vi "rszvl_core_global.vi"() -> ()   [LabVIEW 2014] (continued)
Callback"="", "Coerce Callback"="", "User Callback"="", "Supported Models"="", "Instrument Options"="", "Repeated Capabilities"="", "Restricted Repeated Capabilities"="", "Help"="This attribute configures the R&S FSQ-K91 measurement type to be EVM Versus Carrier. After this command has been executed, the specified measurement will only be started when the user issues the INITiate command.\n\nAvailable Repeated Capabilities:\nNone\n\nRemote-control command(s):\nCONFigure:BURSt:EVM:ECARrier[:IMMediate]", "Flags"={"OPC Wait"=TRUE, "Dont check status"=FALSE, "*WAI"=FALSE}, "Check Status Callback"=""}, {"Level"=3, "Descriptive Name"="WLAN EVM Versus Symbol Measurement", "Class Only"=FALSE, "Data Type"=4, "Access"=1, "Identifier"="RSZVL_ATTR_WLAN_EVM_ESYM", "Range Table"="", "Command"="CONF:BURS:EVM:ESYM", "Read Callback"="", "Write Callback"="", "Range Callback"="", "Check Callback"="", "Rngtable Callback"="", "Coerce Callback"="", "User Callback"="", "Supported Models"="", "Instrument Options"="", "Repeated Capabilities"="", "Restricted Repeated Capabilities"="", "Help"="This attribute configures the FSQ-K91 measurement type to be EVM Versus Symbol. After this command has been executed, the specified measurement will only be started when the user issues the INITiate command\n\nAvailable Repeated Capabilities:\nNone\n\nRemote-control command(s):\nCONFigure:BURSt:EVM:ESYMbol[:IMMediate]", "Flags"={"OPC Wait"=TRUE, "Dont check status"=FALSE, "*WAI"=FALSE}, "Check Status Callback"=""}, {"Level"=3, "Descriptive Name"="WLAN Spectrum MASK", "Class Only"=FALSE, "Data Type"=4, "Access"=1, "Identifier"="RSZVL_ATTR_WLAN_SPEC_MASK", "Range Table"="", "Command"="CONF:BURS:SPEC:MASK", "Read Callback"="", "Write Callback"="", "Range Callback"="", "Check Callback"="", "Rngtable Callback"="", "Coerce Callback"="", "User Callback"="", "Supported Models"="", "Instrument Options"="", "Repeated Capabilities"="", "Restricted Repeated Capabilities"="", "Help"="This attribute configures the R&S FSQ-K91 measurement type to be Spectrum mask. After this command has been executed, the specified measurement will only be started when the user issues the INITiate command\n\nAvailable Repeated Capabilities:\nNone\n\nRemote-control command(s):\nCONFigure:BURSt:SPECtrum:MASK[:IMMediate]", "Flags"={"OPC Wait"=TRUE, "Dont check status"=FALSE, "*WAI"=FALSE}, "Check Status Callback"=""}, {"Level"=3, "Descriptive Name"="WLAN Spectrum MASK Select", "Class Only"=FALSE, "Data Type"=0, "Access"=2, "Identifier"="RSZVL_ATTR_WLAN_SPEC_MASK_SEL", "Range Table"="rszvl_rngSpecMask", "Command"="CONF:BURS:SPEC:MASK:SEL", "Read Callback"="", "Write Callback"="", "Range Callback"="", "Check Callback"="", "Rngtable Callback"="", "Coerce Callback"="", "User Callback"="", "Supported Models"="", "Instrument Options"="", "Repeated Capabilities"="", "Restricted Repeated Capabilities"="", "Help"="This attribute configures how R&S FS-K91 will interpret the Spectrum MASK measurement results.\nThis is either performed using the IEEE or ETSI standard. \n\nNote:\n(1) This attribute is only available for IEEE\n802.11a.\n\nAvailable Repeated Capabilities:\nNone\n\nRemote-control command(s):\nCONFigure:BURSt:SPECtrum:MASK:SELect IEEE | ETSI", "Flags"={"OPC Wait"=FALSE, "Dont check status"=FALSE, "*WAI"=FALSE}, "Check Status Callback"=""}, {"Level"=3, "Descriptive Name"="WLAN Spectrum FFT", "Class Only"=FALSE, "Data Type"=4, "Access"=1, "Identifier"="RSZVL_ATTR_WLAN_SPEC_FFT", "Range Table"="", "Command"="CONF:BURS:SPEC:FFT", "Read Callback"="", "Write Callback"="", "Range Callback"="", "Check Callback"="", "Rngtable Callback"="", "Coerce Callback"="", "User Callback"="", "Supported Models"="", "Instrument Options"="", "Repeated Capabilities"="", "Restricted Repeated Capabilities"="", "Help"="This attribute configures the R&S FSQ-K91 measurement type to be FFT (Fast Fourier Transform). After this command has been executed, the specified measurement will only be started when the user issues the INITiate command\n\nAvailable Repeated Capabilities:\nNone\n\nRemote-control command(s):\nCONFigure:BURSt:SPECtrum:FFT[:IMMediate]", "Flags"={"OPC Wait"=TRUE, "Dont check status"=FALSE, "*WAI"=FALSE}, "Check Status Callback"=""}, {"Level"=3, "Descriptive Name"="WLAN Spectrum ACPR", "Class Only"=FALSE, "Data Type"=4, "Access"=1, "Identifier"="RSZVL_ATTR_WLAN_SPEC_ACPR", "Range Table"="", "Command"="CONF:BURS:SPEC:ACPR", "Read Callback"="", "Write Callback"="", "Range Callback"="", "Check Callback"="", "Rngtable Callback"="", "Coerce Callback"="", "User Callback"="", "Supported Models"="", "Instrument Options"="", "Repeated Capabilities"="", "Restricted Repeated Capabilities"="", "Help"="This attribute configures the R&S FSQ-K91/K92 measurement type to be ACPR (adjacent channel power ratio). After this command has been executed, the specified measurement will only be started when the user issues the INITiate command\n\nAvailable Repeated Capabilities:\nNone\n\nRemote-control command(s):\nCONFigure:BURSt:SPECtrum:ACPR[:IMMediate]", "Flags"={"OPC Wait"=TRUE, "Dont check status"=FALSE, "*WAI"=FALSE}, "Check Status Callback"=""}, {"Level"=3, "Descriptive Name"="WLAN Constelation Versus Symbol", "Class Only"=FALSE, "Data Type"=4, "Access"=1, "Identifier"="RSZVL_ATTR_WLAN_CONS_CSYM", "Range Table"="", "Command"="CONF:BURS:CONS:CSYM", "Read Callback"="", "Write Callback"="", "Range Callback"="", "Check Callback"="", "Rngtable Callback"="", "Coerce Callback"="", "User Callback"="", "Supported Models"="", "Instrument Options"="", "Repeated Capabilities"="", "Restricted Repeated Capabilities"="", "Help"="This attribute configures the R&S FSQ-K91 measurement type to be Constellation versus Symbol. After this command has been executed, the specified measurement will only be started when the user issues the INITiate command\n\nAvailable Repeated Capabilities:\nNone\n\nRemote-control command(s):\nCONFigure:BURSt:CONStellation:CSYMbol[:IMMediate]", "Flags"={"OPC Wait"=TRUE, "Dont check status"=FALSE, "*WAI"=FALSE}, "Check Status Callback"=""}, {"Level"=3, "Descriptive Name"="WLAN Overall Burst Count", "Class Only"=FALSE, "Data Type"=3, "Access"=2, "Identifier"="RSZVL_ATTR_WLAN_BURS_COUN_STAT", "Range Table"="", "Command"="BURS:COUN:STAT", "Read Callback"="", "Write Callback"="", "Range Callback"="", "Check Callback"="", "Rngtable Callback"="", "Coerce Callback"="", "User Callback"="", "Supported Models"="", "Instrument Options"="", "Repeated Capabilities"="", "Restricted Repeated Capabilities"="", "Help"="When this attribute is set to on, the burst count parameter will be used by the measurement,\notherwise the burst count parameter will be ignored.\n\nAvailable Repeated Capabilities:\nNone\n\nRemote-control command(s):\n[SENSe:]BURSt:COUNt:STATe ON | OFF", "Flags"={"OPC Wait"=FALSE, "Dont check status"=FALSE, "*WAI"=FALSE}, "Check Status Callback"=""}, {"Level"=3, "Descriptive Name"="WLAN Constelation Versus Carrier", "Class Only"=FALSE, "Data Type"=4, "Access"=1, "Identifier"="RSZVL_ATTR_WLAN_CONS_CCAR", "Range Table"="", "Command"="CONF:BURS:CONS:CCAR", "Read Callback"="", "Write Callback"="", "Range Callback"="", "Check Callback"="", "Rngtable Callback"="", "Coerce Callback"="", "User Callback"="", "Supported Models"="", "Instrument Options"="", "Repeated Capabilities"="", "Restricted Repeated Capabilities"="", "Help"="This attribute configures the R&S FSQ-K91 measurement type to be Constellation versus Carrier. After this command has been executed, the specified\nmeasurement will only be started when the user issues the INITiate command.\n\nAvailable Repeated Capabilities:\nNone\n\nRemote-control command(s):\nCONFigure:BURSt:CONStellation:CCARrier[:IMMediate]", "Flags"={"OPC Wait"=TRUE, "Dont check status"=FALSE, "*WAI"=FALSE}, "Check Status Callback"=""}, {"Level"=3, "Descriptive Name"="WLAN Constellation Carrier Select", "Class Only"=FALSE, "Data Type"=0, "Access"=2, "Identifier"="RSZVL_ATTR_WLAN_CONS_CARR_SEL", "Range Table"="rszvl_rngBurstSel", "Command"="CONF:BURS:CONS:CARR:SEL", "Read Callback"="", "Write Callback"="", "Range Callback"="", "Check Callback"="", "Rngtable Callback"="", "Coerce Callback"="", "User Callback"="", "Supported Models"="", "Instrument Options"="", "Repeated Capabilities"="", "Restricted Repeated Capabilities"="", "Help"="This attribute is only available when Constellation versus Symbol measurement is selected. When the Constellation versus Symbol measurement is initiated, it will calculate the results of the selected carrier.\n\nNote:\n(1) This attribute is not available for IEEE 802.11b standard.\n\nAvailable Repeated Capabilities:\nNone\n\nRemote-control command(s):\nCONFigure:BURSt:CONStellation:CARRier:SELect ALL | PILOTS", "Flags"={"OPC Wait"=FALSE, "Dont check status"=FALSE, "*WAI"=FALSE}, "Check Status Callback"=""}, {"Level"=3, "Descriptive Name"="WLAN Constellation Carrier Select Num", "Class Only"=FALSE, "Data Type"=0, "Access"=2, "Identifier"="RSZVL_ATTR_WLAN_CONS_CARR_SEL_NR", "Range Table"="", "Command"="CONF:BURS:CONS:CARR:SEL", "Read Callback"="", "Write Callback"="", "Range Callback"="", "Check Callback"="", "Rngtable Callback"="", "Coerce Callback"="", "User Callback"="", "Supported Models"="", "Instrument Options"="", "Repeated Capabilities"="", "Restricted Repeated Capabilities"="", "Help"="This attribute is only available when Constellation versus Symbol measurement is selected. When the Constellation versus Symbol measurement is initiated, it will calculate the results of the selected carrier.\n\nNote:¨\n(1) This attribute is not available for IEEE 802.11b standard.\n\n(2) Values -26 to 26 exclude 0 are available\n\nAvailable Repeated Capabilities:\nNone\n\nRemote-control command(s):\nCONFigure:BURSt:CONStellation:CARRier:SELect nr", "Flags"={"OPC Wait"=FALSE, "Dont check status"=FALSE, "*WAI"=FALSE}, "Check Status Callback"=""}, {"Level"=3, "Descriptive Name"="WLAN Statistics CCDF", "Class Only"=FALSE, "Data Type"=4, "Access"=1, "Identifier"="RSZVL_ATTR_WLAN_STAT_CCDF", "Range Table"="", "Command"="CONF:BURS:STAT:CCDF", "Read Callback"="", "Write Callback"="", "Range Callback"="", "Check Callback"="", "Rngtable Callback"="", "Coerce Callback"="", "User Callback"="", "Supported Models"="", "Instrument Options"="", "Repeated Capabilities"="", "Restricted Repeated Capabilities"="", "Help"="This attribute configures the R&S FSQ-K91 measurement type to be CCDF (conditional cumulative distribution functions.). After this command has been executed, the specified measurement will only be started when the user issues the INITiate command\n\nAvailable Repeated Capabilities:\nNone\n\nRemote-control command(s):\nCONFigure:BURSt:STATistics:CCDF[:IMMediate]", "Flags"={"OPC Wait"=TRUE, "Dont check status"=FALSE, "*WAI"=FALSE}, "Check Status Callback"=""}, {"Level"=3, "Descriptive Name"="WLAN Statistics Bit Stream", "Class Only"=FALSE, "Data Type"=4, "Access"=1, "Identifier"="RSZVL_ATTR_WLAN_STAT_BSTR", "Range Table"="", "Command"="CONF:BURS:STAT:BSTR", "Read Callback"="", "Write Callback"="", "Range Callback"="", "Check Callback"="", "Rngtable Callback"="", "Coerce Callback"="", "User Callback"="", "Supported Models"="", "Instrument Options"="", "Repeated Capabilities"="", "Restricted Repeated Capabilities"="", "Help"="This attribute configures the R&S FSQ-K91 measurement type to be bit stream. After this command has been executed, the specified measurement will only be started when the user issues the INITiate command\n\nAvailable Repeated Capabilities:\nNone\n\nRemote-control command(s):\nCONFigure:BURSt:STATistics:BSTReam[:IMMediate]", "Flags"={"OPC Wait"=TRUE, "Dont check status"=FALSE, "*WAI"=FALSE}, "Check Status Callback"=""}, {"Level"=3, "Descriptive Name"="WLAN Statistics Signal Field", "Class Only"=FALSE, "Data Type"=4, "Access"=1, "Identifier"="RSZVL_ATTR_WLAN_STAT_SFI", "Range Table"="", "Command"="CONF:BURS:STAT:SFI", "Read Callback"="", "Write Callback"="", "Range Callback"="", "Check Callback"="", "Rngtable Callback"="", "Coerce Callback"="", "User Callback"="", "Supported Models"="", "Instrument Options"="", "Repeated Capabilities"="", "Restricted Repeated Capabilities"="", "Help"="This attribute configures the R&S FS-K91 measurement type to be signal field. After this command has been executed, the specified measurement will only be started when the user issues the INITiate command.\n\nAvailable Repeated Capabilities:\nNone\n\nRemote-control command(s):\nCONFigure:BURSt:STATistics:SFIeld [:IMMediate]", "Flags"={"OPC Wait"=TRUE, "Dont check status"=FALSE, "*WAI"=FALSE}, "Check Status Callback"=""}, {"Level"=3, "Descriptive Name"="WLAN Start Measurement", "Class Only"=FALSE, "Data Type"=4, "Access"=1, "Identifier"="RSZVL_ATTR_WLAN_INIT", "Range Table"="", "Command"="INIT", "Read Callback"="", "Write Callback"="", "Range Callback"="", "Check Callback"="", "Rngtable Callback"="", "Coerce Callback"="", "User Callback"="", "Supported Models"="", "Instrument Options"="", "Repeated Capabilities"="", "Restricted Repeated Capabilities"="", "Help"="This attribute requests the R&S FSQ-K91 option to start a new measurement sequence. If a measurement sequence is already in progress, the command will be ignored.\n\nAvailable Repeated Capabilities:\nNone\n\nRemote-control command(s):\nINITiate[:IMMediate]", "Flags"={"OPC Wait"=TRUE, "Dont check status"=FALSE, "*WAI"=FALSE}, "Check Status Callback"=""}, {"Level"=3, "Descriptive Name"="WLAN Run Continuous", "Class Only"=FALSE, "Data Type"=3, "Access"=2, "Identifier"="RSZVL_ATTR_WLAN_INIT_CONT", "Range Table"="", "Command"="INIT:CONT", "Read Callback"="", "Write Callback"="", "Range Callback"="", "Check Callback"="", "Rngtable Callback"="", "Coerce Callback"="", "User Callback"="", "Supported Models"="", "Instrument Options"="", "Repeated Capabilities"="", "Restricted Repeated Capabilities"="", "Help"="This attribute determines whether the trigger system is continuously initiated (continuous) or\nperforms single measurements (single).\n\nAvailable Repeated Capabilities:\nNone\n\nRemote-control command(s):\nINITiate:CONTinuous ON | OFF", "Flags"={"OPC Wait"=FALSE, "Dont check status"=FALSE, "*WAI"=FALSE}, "Check Status Callback"=""}, {"Level"=3, "Descriptive Name"="WLAN Mode", "Class Only"=FALSE, "Data Type"=4, "Access"=1, "Identifier"="RSZVL_ATTR_WLAN_MODE", "Range Table"="", "Command"="INST:SEL WLAN", "Read Callback"="", "Write Callback"="", "Range Callback"="", "Check Callback"="", "Rngtable Callback"="", "Coerce Callback"="", "User Callback"="", "Supported Models"="", "Instrument Options"="", "Repeated Capabilities"="", "Restricted Repeated Capabilities"="", "Help"="This attribute selects active operation of the R&S FSQ-K91 option by specifying its name.\n\nAvailable Repeated Capabilities:\nNone\n\nRemote-control command(s):\nINSTrument:SELect WLAN", "Flags"={"OPC Wait"=FALSE, "Dont check status"=FALSE, "*WAI"=FALSE}, "Check Status Callback"=""}, {"Level"=3, "Descriptive Name"="WLAN Number of Burst", "Class Only"=FALSE, "Data Type"=0, "Access"=2, "Identifier"="RSZVL_ATTR_WLAN_BURS_COUN", "Range Table"="", "Command"="BURS:COUN", "Read Callback"="", "Write Callback"="", "Range Callback"="", "Check Callback"="", "Rngtable Callback"="", "Coerce Callback"="", "User Callback"="", "Supported Models"="", "Instrument Options"="", "Repeated Capabilities"="", "Restricted Repeated Capabilities"="", "Help"="This attribute defines the number of bursts that will be analyzed by the measurement. This attribute is not valid, if the setting for the [SENSe:]BURst:COUNt:STATe parameter is off.\n\nAvailable Repeated Capabilities:\nNone\n\nRemote-control command(s):\n[SENSe:]BURSt:COUNt", "Flags"={"OPC Wait"=FALSE, "Dont check status"=FALSE, "*WAI"=FALSE}, "Check Status Callback"=""}, {"Level"=3, "Descriptive Name"="WLAN Swap IQ", "Class Only"=FALSE, "Data Type"=3, "Access"=2, "Identifier"="RSZVL_ATTR_WLAN_SWAP_IQ", "Range Table"="", "Command"="SWAP", "Read Callback"="", "Write Callback"="", "Range Callback"="", "Check Callback"="", "Rngtable Callback"="", "Coerce Callback"="", "User Callback"="", "Supported Models"="", "Instrument Options"="", "Repeated Capabilities"="", "Restricted Repeated Capabilities"="", "Help"="This attribute defines whether or not the recorded IQ pairs should be swapped (I/Q) before being processed.\n\nAvailable Repeated Capabilities:\nNone\n\nRemote-control command(s):\n[SENSe:]SWAPiq ON|OFF", "Flags"={"OPC Wait"=FALSE, "Dont check status"=FALSE, "*WAI"=FALSE}, "Check Status Callback"=""}, {"Level"=3, "Descriptive Name"="WLAN ACP Mode", "Class Only"=FALSE, "Data Type"=0, "Access"=2, "Identifier"="RSZVL_ATTR_WLAN_ACH_MODE", "Range Table"="rszvl_rngAbsRel", "Command"="POW:ACH:MODE", "Read Callback"="", "Write Callback"="", "Range Callback"="", "Check Callback"="", "Rngtable Callback"="", "Coerce Callback"="", "User Callback"="", "Supported Models"="", "Instrument Options"="", "Repeated Capabilities"="", "Restricted Repeated Capabilities"="", "Help"="This attribut sets the ACP measurement mode to either absolute or relative.\n\nNote:\n(1) This attribute is available only for IEEE 802.11j standard.\n\nAvailable Repeated Capabilities:\nNone\n\nRemote-control command(s):\n[SENSe:]POWer:ACHannel:MODE ABS | REL", "Flags"={"OPC Wait"=FALSE, "Dont check status"=FALSE, "*WAI"=FALSE}, "Check Status Callback"=""}, {"Level"=3, "Descriptive Name"="WLAN Preamble Unit", "Class Only"=FALSE, "Data Type"=0, "Access"=2, "Identifier"="RSZVL_ATTR_WLAN_UNIT_PRE", "Range Table"="rszvl_rngUnitHzPct", "Command"="UNIT:PRE", "Read Callback"="", "Write Callback"="", "Range Callback"="", "Check Callback"="", "Rngtable Callback"="", "Coerce Callback"="", "User Callback"="", "Supported Models"="", "Instrument Options"="", "Repeated Capabilities"="", "Restricted Repeated Capabilities"="", "Help"="This attribute specifies the units for Preamble error results.\n\nAvailable Repeated Capabilities:\nNone\n\nRemote-control command(s):\nUNIT:PREamble HZ | PCT", "Flags"={"OPC Wait"=FALSE, "Dont check status"=FALSE, "*WAI"=FALSE}, "Check Status Callback"=""}, {"Level"=3, "Descriptive Name"="WLAN EVM Unit", "Class Only"=FALSE, "Data Type"=0, "Access"=2, "Identifier"="RSZVL_ATTR_WLAN_UNIT_EVM", "Range Table"="rszvl_rngUnitDbPct", "Command"="UNIT:EVM", "Read Callback"="", "Write Callback"="", "Range Callback"="", "Check Callback"="", "Rngtable Callback"="", "Coerce Callback"="", "User Callback"="", "Supported Models"="", "Instrument Options"="", "Repeated Capabilities"="", "Restricted Repeated Capabilities"="", "Help"="This attribute specifies the units for EVM trace results.\n\nAvailable Repeated Capabilities:\nNone\n\nRemote-control command(s):\nUNIT:EVM DB | PCT", "Flags"={"OPC Wait"=FALSE, "Dont check status"=FALSE, "*WAI"=FALSE}, "Check Status Callback"=""}, {"Level"=3, "Descriptive Name"="WLAN Gain Imbalance Unit", "Class Only"=FALSE, "Data Type"=0, "Access"=2, "Identifier"="RSZVL_ATTR_WLAN_UNIT_GIMB", "Range Table"="rszvl_rngUnitDbPct", "Command"="UNIT:GIMBalance", "Read Callback"="", "Write Callback"="", "Range Callback"="", "Check Callback"="", "Rngtable Callback"="", "Coerce Callback"="", "User Callback"="", "Supported Models"="", "Instrument Options"="", "Repeated Capabilities"="", "Restricted Repeated Capabilities"="", "Help"="This attribute specifies the units for gain imbalance results.\n\nAvailable Repeated Capabilities:\nNone\n\nRemote-control command(s):\nUNIT:GIMBalance DB | PCT", "Flags"={"OPC Wait"=FALSE, "Dont check status"=FALSE, "*WAI"=FALSE}, "Check Status Callback"=""}, {"Level"=3, "Descriptive Name"="WLAN Phase or Frequency vs Preamble", "Class Only"=FALSE, "Data Type"=4, "Access"=1, "Identifier"="RSZVL_ATTR_WLAN_PRE", "Range Table"="", "Command"="CONF:BURS:PRE", "Read Callback"="", "Write Callback"="", "Range Callback"="", "Check Callback"="", "Rngtable Callback"="", "Coerce Callback"="", "User Callback"="", "Supported Models"="", "Instrument Options"="", "Repeated Capabilities"="", "Restricted Repeated Capabilities"="", "Help"="This attribute configures the R&S FSQ-K90/K91 measurement type to be Phase or Frequency Vs Premable. After this command has been executed, the specified measurement will only be started when the user issues the INITiate command\n\nAvailable Repeated Capabilities:\nNone\n\nRemote-control command(s):\nCONFigure:BURSt:PREamble[:IMMediate]", "Flags"={"OPC Wait"=FALSE, "Dont check status"=FALSE, "*WAI"=FALSE}, "Check Status Callback"=""}, {"Level"=3, "Descriptive Name"="WLAN IQ Sample Rate", "Class Only"=FALSE, "Data Type"=1, "Access"=2, "Identifier"="RSZVL_ATTR_WLAN_SRAT", "Range Table"="rszvl_rngIQSRate", "Command"="TRACE:IQ:SRAT", "Read Callback"="", "Write Callback"="", "Range Callback"="", "Check Callback"="", "Rngtable Callback"="", "Coerce Callback"="", "User Callback"="", "Supported Models"="", "Instrument Options"="", "Repeated Capabilities"="", "Restricted Repeated Capabilities"="", "Help"="This attribute allows the sample rate for IQ measurements to be specified. \n\nValid Range: 10.0e3 Hz to 100.0e6 Hz (326.4e6 Hz with option R&S FSQ-B72)\n\nAvailable Repeated Capabilities:\nNone\n\nRemote-control command(s):\nTRACE:IQ:SRATe", "Flags"={"OPC Wait"=FALSE, "Dont check status"=FALSE, "*WAI"=FALSE}, "Check Status Callback"=""}, {"Level"=3, "Descriptive Name"="WLAN Automatic Power Level Sweep Time", "Class Only"=FALSE, "Data Type"=1, "Access"=2, "Identifier"="RSZVL_ATTR_WLAN_POW_AUTO_SWE_TIME", "Range Table"="rszvl_rngAutoLevelTime", "Command"="CONF:POW:AUTO:SWE:TIME", "Read Callback"="", "Write Callback"="", "Range Callback"="", "Check Callback"="", "Rngtable Callback"="", "Coerce Callback"="", "User Callback"="", "Supported Models"="", "Instrument Options"="", "Repeated Capabilities"="", "Restricted Repeated Capabilities"="", "Help"="This attribute specifies the sweep time for the automatic power level detection.\n\nAvailable Repeated Capabilities:\nNone\n\nRemote-control command(s):\nCONFigure:POWer:AUTO:SWEep:TIME", "Flags"={"OPC Wait"=FALSE, "Dont check status"=FALSE, "*WAI"=FALSE}, "Check Status Callback"=""}, {"Level"=3, "Descriptive Name"="WLAN Load IQ Data", "Class Only"=FALSE, "Data Type"=2, "Access"=1, "Identifier"="RSZVL_ATTR_WLAN_IQ_LOAD", "Range Table"="", "Command"="MMEM:LOAD:IQ:STAT", "Read Callback"="", "Write Callback"="rszvl_FileStateSpecialFormat_WriteCallback.vi", "Range Callback"="", "Check Callback"="", "Rngtable Callback"="", "Coerce Callback"="", "User Callback"="", "Supported Models"="", "Instrument Options"="", "Repeated Capabilities"="", "Restricted Repeated Capabilities"="", "Help"="This attribute loads IQ data from the specified .iqw file.\n\nAvailable Repeated Capabilities:\nNone\n\nRemote-control command(s):\nMMEMory:LOAD:IQ:STATe", "Flags"={"OPC Wait"=FALSE, "Dont check status"=FALSE, "*WAI"=FALSE}, "Check Status Callback"=""}, {"Level"=3, "Descriptive Name"="WLAN Save IQ Data", "Class Only"=FALSE, "Data Type"=2, "Access"=1, "Identifier"="RSZVL_ATTR_WLAN_IQ_SAVE", "Range Table"="", "Command"="MMEM:STOR:IQ:STAT", "Read Callback"="", "Write Callback"="rszvl_FileStateSpecialFormat_WriteCallback.vi", "Range Callback"="", "Check Callback"="", "Rngtable Callback"="", "Coerce Callback"="", "User Callback"="", "Supported Models"="", "Instrument Options"="", "Repeated Capabilities"="", "Restricted Repeated Capabilities"="", "Help"="This attribute stores IQ data to the specified .iqw file.\n\nAvailable Repeated Capabilities:\nNone\n\nRemote-control command(s):\nMMEMory:STORe:IQ:STATe", "Flags"={"OPC Wait"=FALSE, "Dont check status"=FALSE, "*WAI"=FALSE}, "Check Status Callback"=""}, {"Level"=3, "Descriptive Name"="WLAN Burst Recalculate", "Class Only"=FALSE, "Data Type"=4, "Access"=1, "Identifier"="RSZVL_ATTR_WLAN_CALC_BURS", "Range Table"="", "Command"="CALC:BURS", "Read Callback"="", "Write Callback"="", "Range Callback"="", "Check Callback"="", "Rngtable Callback"="", "Coerce Callback"="", "User Callback"="", "Supported Models"="", "Instrument Options"="", "Repeated Capabilities"="", "Restricted Repeated Capabilities"="", "Help"="This attribute forces the IQ measurement results to be recalculated according to the current settings\n\nAvailable Repeated Capabilities:\nNone\n\nRemote-control command(s):\nCALCulate<1|2>:BURSt[:IMMediate]", "Flags"={"OPC Wait"=FALSE, "Dont check status"=FALSE, "*WAI"=FALSE}, "Check Status Callback"=""}, {"Level"=3, "Descriptive Name"="WLAN Preamble Select", "Class Only"=FALSE, "Data Type"=0, "Access"=2, "Identifier"="RSZVL_ATTR_WLAN_PRE_SEL", "Range Table"="rszvl_rngPreamble", "Command"="CONF:BURS:PRE:SEL", "Read Callback"="", "Write Callback"="", "Range Callback"="", "Check Callback"="", "Rngtable Callback"="", "Coerce Callback"="", "User Callback"="", "Supported Models"="", "Instrument Options"="", "Repeated Capabilities"="", "Restricted Repeated Capabilities"="", "Help"="This attribute specifies whether Frequency or Phase results are displayed when the\nmeasurement type is set to Error Vs Preamble\n\nAvailable Repeated Capabilities:\nNone\n\nRemote-control command(s):\nCONFigure:BURSt:PREamble:SELect FREQ | PHASe", "Flags"={"OPC Wait"=FALSE, "Dont check status"=FALSE, "*WAI"=FALSE}, "Check Status Callback"=""}, {"Level"=2, "Descriptive Name"="Display", "Class Only"=TRUE, "Data Type"=0, "Access"=0, "Identifier"="", "Range Table"="", "Command"="", "Read Callback"="", "Write Callback"="", "Range Callback"="", "Check Callback"="", "Rngtable Callback"="", "Coerce Callback"="", "User Callback"="", "Supported Models"="", "Instrument Options"="", "Repeated Capabilities"="", "Restricted Repeated Capabilities"="", "Help"="Attributes that configure the display.\n\n(1) WLAN Display Table:\nThis attribute selects whether the results table is displayed.\n\n(2) WLAN Y Axis Auto Scaling:\nThis attribute switches on or off automatic scaling of the Y-axis for the specified trace display. Automatic scaling sets the Y-axis to automatically scale to best fit the measurement results. \n\nNote:\n(1) This attribute is only available for the following result displays:\nEVM vs Carrier\nEVM vs Symbol\nFrequency error vs Preamble\nPhase error vs Preamble\n\n\n(3) WLAN Y Scale Division:\nThis attribute sets the size of each Y scale division for the specified trace display. \n\nNote:\n(1) This attribute has no affect if automatic scaling of the Y-axis is enabled. \n\n(2) This attribute is only available for\nthe following result displays:\nEVM vs Carrier\nEVM vs Symbol\nFrequency error vs Preamble\nPhase error vs Preamble", "Flags"={"OPC Wait"=FALSE, "Dont check status"=FALSE, "*WAI"=FALSE}, "Check Status Callback"=""}, {"Level"=3, "Descriptive Name"="WLAN Display Table", "Class Only"=FALSE, "Data Type"=3, "Access"=2, "Identifier"="RSZVL_ATTR_WLAN_DISP_TABL", "Range Table"="", "Command"="DISP:WIND:TABL", "Read Callback"="", "Write Callback"="", "Range Callback"="", "Check Callback"="", "Rngtable Callback"="", "Coerce Callback"="", "User Callback"="", "Supported Models"="", "Instrument Options"="", "Repeated Capabilities"="", "Restricted Repeated Capabilities"="", "Help"="This attribute selects whether the results table is displayed.\n\nAvailable Repeated Capabilities:\nNone\n\nRemote-control command(s):\nDISPlay[:WINDow<1|2>]:TABLe ON | OFF", "Flags"={"OPC Wait"=FALSE, "Dont check status"=FALSE, "*WAI"=FALSE}, "Check Status Callback"=""}, {"Level"=3, "Descriptive Name"="WLAN Screen Select", "Class Only"=FALSE, "Data Type"=4, "Access"=1, "Identifier"="RSZVL_ATTR_WLAN_SCREEN_SELECT", "Range Table"="", "Command"="DISP:WIND{Window}:SSEL", "Read Callback"="", "Write Callback"="", "Range Callback"="", "Check Callback"="", "Rngtable Callback"="", "Coerce Callback"="", "User Callback"="", "Supported Models"="", "Instrument Options"="", "Repeated Capabilities"="", "Restricted Repeated Capabilities"="", "Help"="This attribute selects whether screen A or screen B is active. SSELect means Screen SELect.\n\nAvailable Repeated Capabilities:\nWindow: Win1,Win2\r\n\nRemote-control command(s):\nDISPlay[:WINDow<1|2>]:SSELect", "Flags"={"OPC Wait"=FALSE, "Dont check status"=FALSE, "*WAI"=FALSE}, "Check Status Callback"=""}, {"Level"=3, "Descriptive Name"="WLAN Display Format", "Class Only"=FALSE, "Data Type"=0, "Access"=2, "Identifier"="RSZVL_ATTR_WLAN_DISP_FORMAT", "Range Table"="rszvl_rngDISPFormat", "Command"="DISP:FORM", "Read Callback"="", "Write Callback"="", "Range Callback"="", "Check Callback"="", "Rngtable Callback"="", "Coerce Callback"="", "User Callback"="", "Supported Models"="", "Instrument Options"="", "Repeated Capabilities"="", "Restricted Repeated Capabilities"="", "Help"="This attribute sets the visible screen display type to full or split screen.\n\nAvailable Repeated Capabilities:\nNone\n\nRemote-control command(s):\nDISPlay:FORMat SINGle | SPLit", "Flags"={"OPC Wait"=FALSE, "Dont check status"=FALSE, "*WAI"=FALSE}, "Check Status Callback"=""}, {"Level"=3, "Descriptive Name"="WLAN Y Axis Auto Scaling", "Class Only"=FALSE, "Data Type"=3, "Access"=2, "Identifier"="RSZVL_ATTR_WLAN_DISP_AUTO_Y", "Range Table"="", "Command"="DISP:WIND{Window}:TRAC{Trace}:Y:AUTO", "Read Callback"="", "Write Callback"="", "Range Callback"="", "Check Callback"="", "Rngtable Callback"="", "Coerce Callback"="", "User Callback"="", "Supported Models"="", "Instrument Options"="", "Repeated Capabilities"="", "Restricted Repeated Capabilities"="", "Help"="This attribute switches on or off automatic scaling of the Y-axis for the specified trace display. Automatic scaling sets the Y-axis to automatically scale to best fit the measurement results. \n\nNote:\n(1) This attribute is only available for the following result displays:\nEVM vs Carrier\nEVM vs Symbol\nFrequency error vs Preamble\nPhase error vs Preamble\n\nAvailable Repeated Capabilities:\nWindow: Win1,Win2\r\nTrace: TR1,TR2,TR3,TR4,TR5,TR6,TR7,TR8,TR9,TR10,TR11,TR12,TR13,TR14,TR15,TR16,TR17,TR18,TR19,TR20\r\n\nRemote-control command(s):\nDISPlay[:WINDow<1|2>]:TRACe<1…3>:Y[:SCALe]:AUTO", "Flags"={"OPC Wait"=FALSE, "Dont check status"=FALSE, "*WAI"=FALSE}, "Check Status Callback"=""}, {"Level"=3, "Descriptive Name"="WLAN Y Scale Division", "Class Only"=FALSE, "Data Type"=1, "Access"=2, "Identifier"="RSZVL_ATTR_WLAN_Y_PDIV", "Range Table"="", "Command"="DISP:WIND{Window}:TRAC{Trace}:Y:PDIV", "Read Callback"="", "Write Callback"="", "Range Callback"="", "Check Callback"="", "Rngtable Callback"="", "Coerce Callback"="", "User Callback"="", "Supported Models"="", "Instrument Options"="", "Repeated Capabilities"="", "Restricted Repeated Capabilities"="", "Help"="This attribute sets the size of each Y scale division for the specified trace display. \n\nNote:\n(1) This attribute has no affect if automatic scaling of the Y-axis is enabled. \n\n(2) This attribute is only available for\nthe following result displays:\nEVM vs Carrier\nEVM vs Symbol\nFrequency error vs Preamble\nPhase error vs Preamble\n\nAvailable Repeated Capabilities:\nWindow: Win1,Win2\r\nTrace: TR1,TR2,TR3,TR4,TR5,TR6,TR7,TR8,TR9,TR10,TR11,TR12,TR13,TR14,TR15,TR16,TR17,TR18,TR19,TR20\r\n\nRemote-control command(s):\nDISPlay[:WINDow<1|2>]:TRACe<1…3>:Y[:SCALe]:PDIVision", "Flags"={"OPC Wait"=FALSE, "Dont check status"=FALSE, "*WAI"=FALSE}, "Check Status Callback"=""}, {"Level"=2, "Descriptive Name"="Limit Settings", "Class Only"=TRUE, "Data Type"=0, "Access"=0, "Identifier"="", "Range Table"="", "Command"="", "Read Callback"="", "Write Callback"="", "Range Callback"="", "Check Callback"="", "Rngtable Callback"="", "Coerce Callback"="", "User Callback"="", "Supported Models"="", "Instrument Options"="", "Repeated Capabilities"="", "Restricted Repeated Capabilities"="", "Help"="Attributes that configure the limit settings.\n\n(1) WLAN Rise Time Limit:\nThis attribute sets the rise time limit in seconds\n\nNote:\n(1) This attribute is valid only if standard IEEE 802.11b is selected.\n\n(2) WLAN Fall Time Limit:\nThis attribute sets the fall time limit in seconds\n\nNote:\n(1) This attribute is valid only if standard IEEE 802.11b is selected.\n\n(3) WLAN Frequency Error Limit:\nThis attribute sets the frequency error limit in Hz.\n\n(4) WLAN Symbol Error Limit:\nThis attribute sets the symbol error limit in Hz.\n\n(5) WLAN IQ Offset Error Limit:\nThis attribute sets the IQ Offset error limit in dB.\n\n(6) WLAN EVM Limit:\nThis attribute sets the Error Vector Magnitude Limit in dB.\n\nNote:\n(1) This attribute is available only for the IEEE 802.11b standard.\n\n(7) WLAN Combined EVM Limit:\nThis attribute sets the Error Vector Magnitude Limit in dB. This is a combined figure that represents the pilot, data and the free carrier.\n\n(8) WLAN Data Carrier EVM Limit:\nThis attribute sets the Error Vector Magnitude limit summary for the data carrier in dB.\n\n(9) WLAN Pilot Carrier EVM Limit:\nThis attribute sets the Error Vector Magnitude limit summary for the pilot carriers in dB.", "Flags"={"OPC Wait"=FALSE, "Dont check status"=FALSE, "*WAI"=FALSE}, "Check Status Callback"=""}, {"Level"=3, "Descriptive Name"="WLAN Rise Time Limit", "Class Only"=FALSE, "Data Type"=1, "Access"=2, "Identifier"="RSZVL_ATTR_WLAN_TRIS", "Range Table"="", "Command"="CALC{Window}:LIM{Limit}:BURS:TRIS:{ModifMinMaxAver}", "Read Callback"="", "Write Callback"="", "Range Callback"="", "Check Callback"="", "Rngtable Callback"="", "Coerce Callback"="", "User Callback"="", "Supported Models"="", "Instrument Options"="", "Repeated Capabilities"="", "Restricted Repeated Capabilities"="", "Help"="This attribute sets the rise time limit in seconds\n\nNote:\n(1) This attribute is valid only if standard IEEE 802.11b is selected.\n\nAvailable Repeated Capabilities:\nWindow: Win1,Win2\r\nLimit: L1,L2,L3,L4,L5,L6,L7,L8\r\nModifMinMaxAver: Min,Max,Aver\r\n\nRemote-control command(s):\nCALCulate<1|2>:LIMit<1>:BURSt:TRISe<[:AVERage] | :MAXimum>", "Flags"={"OPC Wait"=FALSE, "Dont check status"=FALSE, "*WAI"=FALSE}, "Check Status Callback"=""}, {"Level"=3, "Descriptive Name"="WLAN Fall Time Limit", "Class Only"=FALSE, "Data Type"=1, "Access"=2, "Identifier"="RSZVL_ATTR_WLAN_TFAL", "Range Table"="", "Command"="CALC{Window}:LIM{Limit}:BURS:TFAL:{ModifMinMaxAver}", "Read Callback"="", "Write Callback"="", "Range Callback"="", "Check Callback"="", "Rngtable Callback"="", "Coerce Callback"="", "User Callback"="", "Supported Models"="", "Instrument Options"="", "Repeated Capabilities"="", "Restricted Repeated Capabilities"="", "Help"="This attribute sets the fall time limit in seconds\n\nNote:\n(1) This attribute is valid only if standard IEEE 802.11b is selected.\n\nAvailable Repeated Capabilities:\nWindow: Win1,Win2\r\nLimit: L1,L2,L3,L4,L5,L6,L7,L8\r\nModifMinMaxAver: Min,Max,Aver\r\n\nRemote-control command(s):\nCALCulate<1|2>:LIMit<1>:BURSt:TFALl<[:AVERage] | :MAXimum>", "Flags"={"OPC Wait"=FALSE, "Dont check status"=FALSE, "*WAI"=FALSE}, "Check Status Callback"=""}, {"Level"=3, "Descriptive Name"="WLAN Frequency Error Limit", "Class Only"=FALSE, "Data Type"=1, "Access"=2, "Identifier"="RSZVL_ATTR_WLAN_FERR", "Range Table"="", "Command"="CALC{Window}:LIM{Limit}:BURS:FERR:{ModifMinMaxAver}", "Read Callback"="", "Write Callback"="", "Range Callback"="", "Check Callback"="", "Rngtable Callback"="", "Coerce Callback"="", "User Callback"="", "Supported Models"="", "Instrument Options"="", "Repeated Capabilities"="", "Restricted Repeated Capabilities"="", "Help"="This attribute sets the frequency error limit in Hz.\n\nAvailable Repeated Capabilities:\nWindow: Win1,Win2\r\nLimit: L1,L2,L3,L4,L5,L6,L7,L8\r\nModifMinMaxAver: Min,Max,Aver\r\n\nRemote-control command(s):\nCALCulate<1|2>:LIMit<1>:BURSt:FERRor<[:AVERage] | :MAXimum>", "Flags"={"OPC Wait"=FALSE, "Dont check status"=FALSE, "*WAI"=FALSE}, "Check Status Callback"=""}, {"Level"=3, "Descriptive Name"="WLAN Symbol Error Limit", "Class Only"=FALSE, "Data Type"=1, "Access"=2, "Identifier"="RSZVL_ATTR_WLAN_SYMB", "Range Table"="", "Command"="CALC{Window}:LIM{Limit}:BURS:SYMB:{ModifMinMaxAver}", "Read Callback"="", "Write Callback"="", "Range Callback"="", "Check Callback"="", "Rngtable Callback"="", "Coerce Callback"="", "User Callback"="", "Supported Models"="", "Instrument Options"="", "Repeated Capabilities"="", "Restricted Repeated Capabilities"="", "Help"="This attribute sets the symbol error limit in Hz.\n\nAvailable Repeated Capabilities:\nWindow: Win1,Win2\r\nLimit: L1,L2,L3,L4,L5,L6,L7,L8\r\nModifMinMaxAver: Min,Max,Aver\r\n\nRemote-control command(s):\nCALCulate<1|2>:LIMit<1>:BURSt:SYMBolerror<[:AVERage] | :MAXimum>", "Flags"={"OPC Wait"=FALSE, "Dont check status"=FALSE, "*WAI"=FALSE}, "Check Status Callback"=""}, {"Level"=3, "Descriptive Name"="WLAN IQ Offset Error Limit", "Class Only"=FALSE, "Data Type"=1, "Access"=2, "Identifier"="RSZVL_ATTR_WLAN_IQOF", "Range Table"="", "Command"="CALC{Window}:LIM{Limit}:BURS:IQOF:{ModifMinMaxAver}", "Read Callback"="", "Write Callback"="", "Range Callback"="", "Check Callback"="", "Rngtable Callback"="", "Coerce Callback"="", "User Callback"="", "Supported Models"="", "Instrument Options"="", "Repeated Capabilities"="", "Restricted Repeated Capabilities"="", "Help"="This attribute sets the IQ Offset error limit in dB.\n\nAvailable Repeated Capabilities:\nWindow: Win1,Win2\r\nLimit: L1,L2,L3,L4,L5,L6,L7,L8\r\nModifMinMaxAver: Min,Max,Aver\r\n\nRemote-control command(s):\nCALCulate<1|2>:LIMit<1>:BURSt:IQOFfset<[:AVERage] | :MAXimum>", "Flags"={"OPC Wait"=FALSE, "Dont check status"=FALSE, "*WAI"=FALSE}, "Check Status Callback"=""}, {"Level"=3, "Descriptive Name"="WLAN EVM Limit", "Class Only"=FALSE, "Data Type"=1, "Access"=2, "Identifier"="RSZVL_ATTR_WLAN_EVM", "Range Table"="", "Command"="CALC{Window}:LIM{Limit}:BURS:EVM:{ModifMinMaxAver}", "Read Callback"="", "Write Callback"="", "Range Callback"="", "Check Callback"="", "Rngtable Callback"="", "Coerce Callback"="", "User Callback"="", "Supported Models"="", "Instrument Options"="", "Repeated Capabilities"="", "Restricted Repeated Capabilities"="", "Help"="This attribute sets the Error Vector Magnitude Limit in dB.\n\nNote:\n(1) This attribute is available only for the IEEE 802.11b standard.\n\nAvailable Repeated Capabilities:\nWindow: Win1,Win2\r\nLimit: L1,L2,L3,L4,L5,L6,L7,L8\r\nModifMinMaxAver: Min,Max,Aver\r\n\nRemote-control command(s):\nCALCulate<1|2>:LIMit<1>:BURSt:EVM<[:AVERage] | :MAXimum>", "Flags"={"OPC Wait"=FALSE, "Dont check status"=FALSE, "*WAI"=FALSE}, "Check Status Callback"=""}, {"Level"=3, "Descriptive Name"="WLAN Combined EVM Limit", "Class Only"=FALSE, "Data Type"=1, "Access"=2, "Identifier"="RSZVL_ATTR_WLAN_EVM_ALL", "Range Table"="", "Command"="CALC{Window}:LIM{Limit}:BURS:EVM:ALL:{ModifMinMaxAver}", "Read Callback"="", "Write Callback"="", "Range Callback"="", "Check Callback"="", "Rngtable Callback"="", "Coerce Callback"="", "User Callback"="", "Supported Models"="", "Instrument Options"="", "Repeated Capabilities"="", "Restricted Repeated Capabilities"="", "Help"="This attribute sets the Error Vector Magnitude Limit in dB. This is a combined figure that represents the pilot, data and the free carrier.\n\nAvailable Repeated Capabilities:\nWindow: Win1,Win2\r\nLimit: L1,L2,L3,L4,L5,L6,L7,L8\r\nModifMinMaxAver: Min,Max,Aver\r\n\nRemote-control command(s):\nCALCulate<1|2>:LIMit<1>:BURSt:EVM:ALL<[:AVERage] | :MAXimum>", "Flags"={"OPC Wait"=FALSE, "Dont check status"=FALSE, "*WAI"=FALSE}, "Check Status Callback"=""}, {"Level"=3, "Descriptive Name"="WLAN Data Carrier EVM Limit", "Class Only"=FALSE, "Data Type"=1, "Access"=2, "Identifier"="RSZVL_ATTR_WLAN_EVM_DATA", "Range Table"="", "Command"="CALC{Window}:LIM{Limit}:BURS:EVM:DATA:{ModifMinMaxAver}", "Read Callback"="", "Write Callback"="", "Range Callback"="", "Check Callback"="", "Rngtable Callback"="", "Coerce Callback"="", "User Callback"="", "Supported Models"="", "Instrument Options"="", "Repeated Capabilities"="", "Restricted Repeated Capabilities"="", "Help"="This attribute sets the Error Vector Magnitude limit summary for the data carrier in dB.\n\nAvailable Repeated Capabilities:\nWindow: Win1,Win2\r\nLimit: L1,L2,L3,L4,L5,L6,L7,
